vi "GCode_Class1_Dynamic1.vi"(8 "error in (no error)":errorcluster, 11 "GCode_Class1 in":refnum<class "GCode_New_ClassName.lvclass">) -> (0 "error out":errorcluster, 3 "GCode_Class1 out":refnum<class "GCode_New_ClassName.lvclass">)   [LabVIEW 2013, in "GCode_New_ClassName.lvclass"]
uses:
  GCode_New_ClassName.lvclass
panel:
  in  "Numeric":dbl
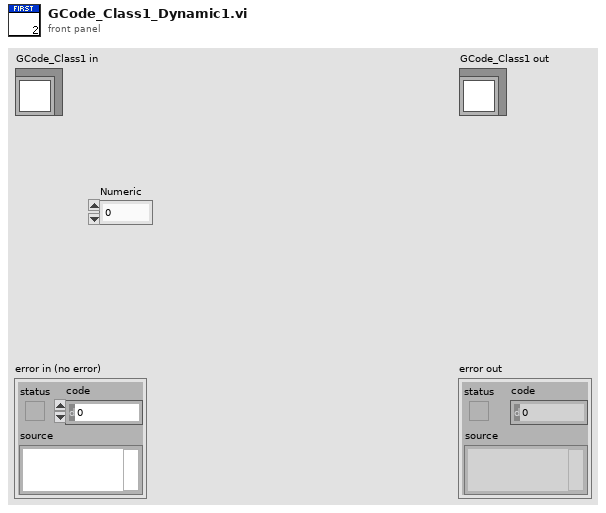
[diagram p1: front panel]
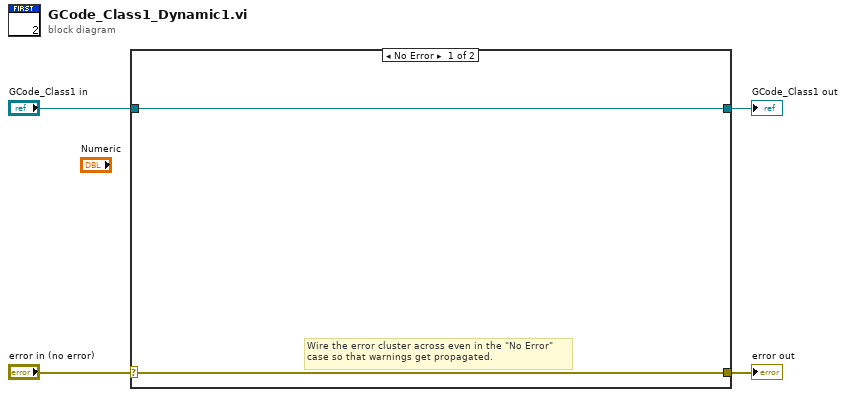
[diagram p0: block diagram]
diagram:
  n1 = case shown="No Error" "error in (no error)" {
    selector: "error in (no error)" -> [w5 w8]
    tunnel: [w5 w8] -> w3
    tunnel: [w6 w7] -> w1
    tunnel: "GCode_Class1 in" -> [w6 w7]
    frame No Error {
      # "Wire the error cluster across even in the \"No Error\"\ncase so that warnings get propagated."
    }
    frame Error {
    }
  }
  "error out" <- w3
  "GCode_Class1 out" <- w1
